vi "initializer_prepare_specfile.vi"(8 "error in (no error)":errorcluster, 10 "appended path":path, 11 "TreeControl in":refnum<vi>) -> ()   [LabVIEW 2019]
uses:
  lib/libSpecValiReader/libSpecValiReader.lvlib
  lib/libSimulationControl/libSimulationControl.lvlib
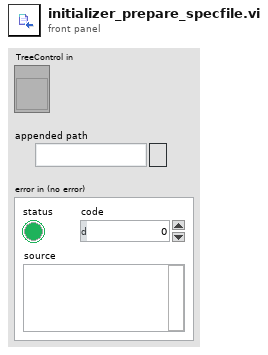
[diagram p1: front panel]
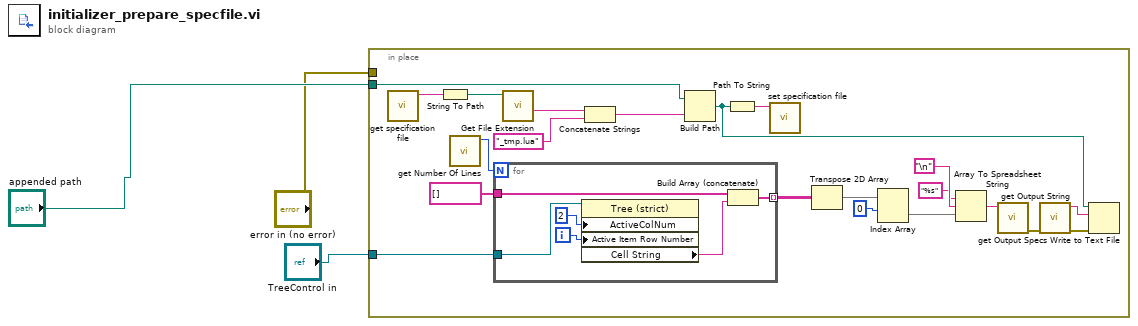
[diagram p0: block diagram]
diagram:
  n1 = in-place {
    in-place-border: "error in (no error)" -> [_]
    in-place-border: "appended path" -> [w11]
    in-place-border: "TreeControl in" -> [w4]
    n2 = call "get specification file.vi"() -> ("function return"=w12:string)  [unwired: 10 in, 1 out]
    n3 = String To Path(string=w12) -> (path=w6:path)
    n4 = call "get Number Of Lines.vi"() -> ("function return"=w16:i32)  [unwired: 10 in, 1 out]
    n5 = for {
      N: w16 -> [_]
      tunnel: string[] [] ("Empty Val Arr") -> [w28]
      tunnel: [w27] -> w21 mode=indexing
      tunnel: w4 -> [w25]
      i -> [w30]
      n6 = property on="Property Node" class="Tree (strict)"(reference=w25, "ActiveColNum"=2 ("Active Cell:Active Column Number"), "Active Item Row Number"=w30) -> ("Cell String"=w26:string)  [unwired: 1 in, 2 out]
      n7 = Build Array (concatenate)(w28, w26) -> (w27:string[])
    }
    n8 = call <vilib>:"Get File Extension.vi"("file"=w6) -> ("filename without extension"=w5:string)  [unwired: 6 in, 4 out]
    n9 = Concatenate Strings(w5, "_tmp.lua" ("string")) -> (w9:string)
    n10 = Build Path(base path=w11, name or relative path=w9) -> (appended path=w8:path)
    n11 = Path To String(path=w8) -> (string=w7:string)
    n12 = call "set specification file.vi"("spec_file"=w7) -> ()  [unwired: 10 in, 1 out]
    n13 = Transpose 2D Array(2D array=w21) -> (transposed array=w22:string[][])
    n14 = Index Array(array=w22, index (row)=0) -> (element=w23:string[])  [unwired: 1 in]
    n15 = Array To Spreadsheet String(delimiter (Tab)="\n", array=w23, 3:"%s" ("format string")) -> (spreadsheet string=w24:string)
    n16 = call "get Output Specs.vi"("specs"=w24) -> ("error out"=w15:errorcluster)  [unwired: 9 in, 1 out]
    n17 = call "get Output String.vi"("error in (no error)"=w15) -> ("error out"=w14:errorcluster, "function return"=w13:string)  [unwired: 9 in]
    n18 = Write to Text File(file (use dialog)=w8, text=w13, error in=w14) -> ()  [unwired: 1 in, 3 out]
  }
